vi "test_Remove Local Chassis.vi"(8 "error in (no error)":errorcluster, 11 "TestCase in":refnum<class "Scan Engine Scripting API Custom Device Unit Tests.lvclass">) -> (0 "error out":errorcluster, 3 "TestCase out":refnum<class "Scan Engine Scripting API Custom Device Unit Tests.lvclass">)   [LabVIEW 2020, in "Scan Engine Scripting API Custom Device Unit Tests.lvclass"]
uses:
  Scan Engine Scripting API Custom Device Unit Tests.lvclass
  Shared/Type Defs/Main Settings.ctl
  Shared/Type Defs/Local Chassis Settings.ctl
  Scan Engine Scripting API Custom Device Unit Tests.lvclass/Scan Engine Scripting API Custom Device Unit Tests.ctl
  <vilib>/addons/_JKI Toolkits/VI Tester/TestCase.llb/TestCase.lvclass
  Scripting/Scan Engine Scripting.lvlib
  Shared/SEECD Shared.lvlib
  C:/Program Files (x86)/National Instruments/LabVIEW 2020/vi.lib/addons/_JKI Toolkits/VI Tester/TestCase.llb/TestCase.lvclass
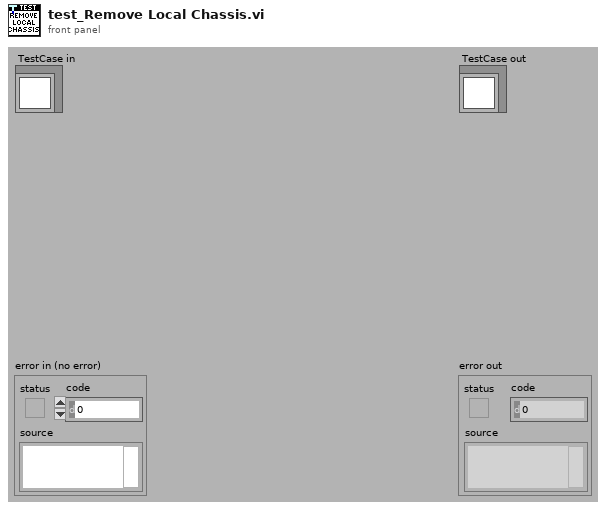
[diagram p1: front panel]
types:
  T1 = typedef "SEECD Shared.lvlib/Local Chassis Settings.ctl" = cluster{"name":string, "number of slots":i32}
  T2 = typedef "SEECD Shared.lvlib/Main Settings.ctl" = cluster{"sync to scan":bool, "scan engine decimation":u16, "delay after FPGA load (s)":u16}
  T3 = typedef "Custom Device API.lvlib/Custom Device Item Ref.ctl" = u64
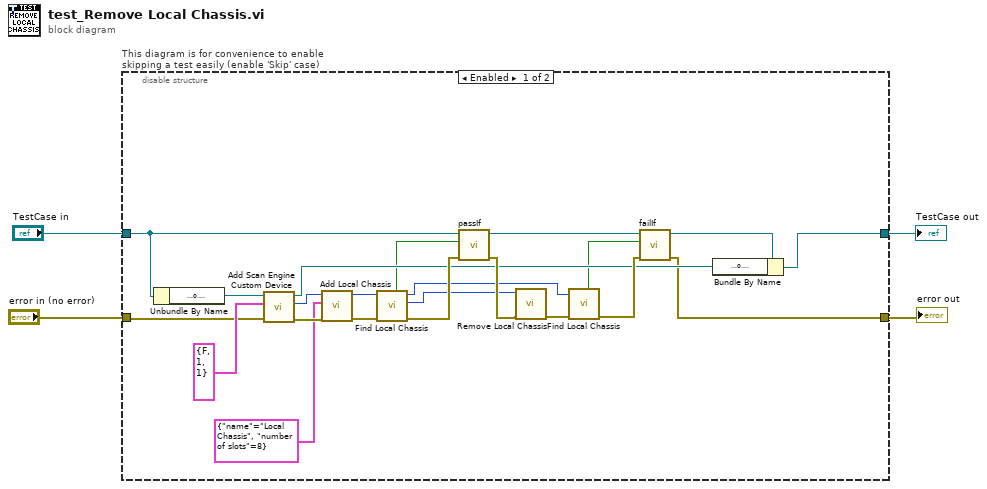
[diagram p0: block diagram]
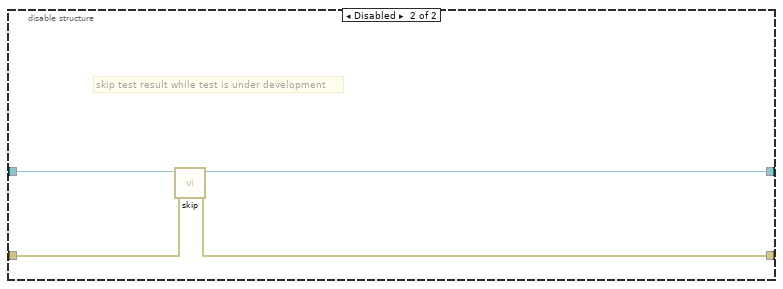
[diagram p2: hidden frame]
diagram:
  n1 = disable-structure "This diagram is for convenience to enable skipping a test easily (enable 'Skip' case)" shown="Enabled" {
    disable-tunnel: "TestCase in" -> [w13 w30]
    disable-tunnel: [w9 w28] -> w1
    disable-tunnel: [w7 w29] -> w3
    disable-tunnel: "error in (no error)" -> [w11 w27]
    frame Enabled {
      n2 = Unbundle By Name(w13) -> ("target ref"=w12:refnum<k24>)
      n3 = call "Add Scan Engine Custom Device.vi"("error in"=w11, "settings"=T2 {"sync to scan"=FALSE, "scan engine decimation"=1, "delay after FPGA load (s)"=1}, "target in"=w12) -> ("error out"=w23:errorcluster, "scan engine custom device ref"=w24:T3, "target out"=w8:refnum<k24>)  [unwired: 6 in]
      n4 = call "Add Local Chassis.vi"("error in"=w23, "settings"=T1 {"name"="Local Chassis", "number of slots"=8}, "scan engine custom device ref in"=w24) -> ("error out"=w21:errorcluster, "scan engine custom device ref out"=w17:T3)  [unwired: 4 in, 3 out]
      n5 = call "Find Local Chassis.vi"("error in"=w21, "scan engine custom device ref in"=w17) -> ("error out"=w19:errorcluster, "local chassis ref"=w16:T3, "scan engine custom device ref out"=w15:T3, "found"=w6:bool)  [unwired: 4 in, 2 out]
      n6 = call-dynamic "passIf.vi"("error in (no error)"=w19, "pass"=w6, "TestCase in"=w13) -> ("error out"=w20:errorcluster, "TestCase out"=w25:refnum<class "Scan Engine Scripting API Custom Device Unit Tests.lvclass">)  [unwired: 7 in]
      n7 = call "Remove Local Chassis.vi"("error in"=w20, "local chassis ref"=w16) -> ("error out"=w18:errorcluster)  [unwired: 9 in]
      n8 = call "Find Local Chassis.vi"("error in"=w18, "scan engine custom device ref in"=w15) -> ("error out"=w14:errorcluster, "found"=w5:bool)  [unwired: 4 in, 4 out]
      n9 = call-dynamic "failIf.vi"("error in (no error)"=w14, "fail"=w5, "TestCase in"=w25) -> ("error out"=w7:errorcluster, "TestCase out"=w10:refnum<class "Scan Engine Scripting API Custom Device Unit Tests.lvclass">)  [unwired: 7 in]
      n10 = Bundle By Name(cluster=w10, "target ref"=w8) -> (w9:refnum<class "Scan Engine Scripting API Custom Device Unit Tests.lvclass">)
    }
    frame Disabled {
      # "skip test result while test is under development"
      n11 = call <vilib>:"skip.vi"("error in (no error)"=w27, "TestCase in"=w30) -> ("error out"=w29:errorcluster, "TestCase out"=w28:refnum<class "Scan Engine Scripting API Custom Device Unit Tests.lvclass">)  [unwired: 8 in]
    }
  }
  "error out" <- w3
  "TestCase out" <- w1
